vi "例4-30.vi"() -> ()   [LabVIEW 2019]
panel:
  out "XY图":cluster{cluster{dbl, dbl}[]}[](graph)
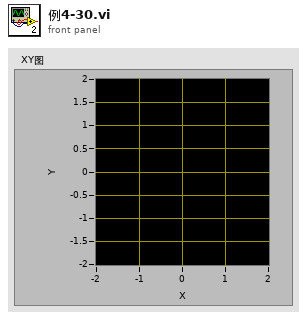
[diagram p1: front panel]
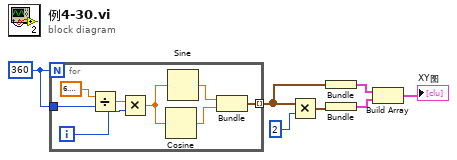
[diagram p0: block diagram]
diagram:
  w7 = 360
  n1 = for {
    N: w7 -> [_]
    tunnel: w7 -> [w14]
    tunnel: [w9] -> w6 mode=indexing
    i -> [w8]
    n2 = Divide(x=6.283185307179586, y=w14) -> (x/y=w13:dbl)
    n3 = Multiply(x=w13, y=w8) -> (x*y=w12:dbl)
    n4 = Cosine(x=w12) -> (cos(x)=w10:dbl)
    n5 = Sine(x=w12) -> (sin(x)=w11:dbl)
    n6 = Bundle(w11, w10) -> (w9:cluster{dbl, dbl})  [unwired: 1 in]
  }
  n7 = Multiply(x=w6, y=2) -> (x*y=w4:cluster{dbl, dbl}[])
  n8 = Bundle(w6) -> (w3:cluster{cluster{dbl, dbl}[]})  [unwired: 1 in]
  n9 = Bundle(w4) -> (w2:cluster{cluster{dbl, dbl}[]})  [unwired: 1 in]
  n10 = Build Array(w3, w2) -> (→"XY图":cluster{cluster{dbl, dbl}[]}[])
